vi "Opt3.vi"(0 "Activation Function":enum32{"Sigmoid", "RELU", "Tanh", "Leaky RELU"}(ring), 1 "Weights l+1":dbl[][](array[numeric]), 2 "Weights":dbl[][](array[numeric]), 3 "Biases":dbl[](array[numeric]), 5 "Net Output":dbl[](array[numeric]), 7 "Activations l-1":dbl[](array[numeric]) format="%.2f", 9 "Delta l+1":dbl[](array[numeric]), 12 "Weight Regularizers":enum32{"None", "L1", "L2"}(radio), 13 "Adam Data In":T1) -> (6 "Updated Weights":dbl[][](array[numeric]), 8 "Updated Biases":dbl[](array[numeric]), 14 "Adam Data Out":T1)   [LabVIEW 2019]
uses:
  Iteration Counter.vi
  <vilib>/Analysis/NI_AALBase.lvlib
  <vilib>/Analysis/Matrix/NI_Matrix.lvlib
  <vilib>/Analysis/Matrix/Numeric/Conversions/Matrix To Array - RM.vi
  <vilib>/Analysis/baseanly.llb/Real Outer Product.vi
  <vilib>/Analysis/baseanly.llb/A x Vector.vi
  Adam_data.ctl
panel:
  out "Grad. w":dbl[][](array[numeric])
  out "Grad. b":dbl[](array[numeric])
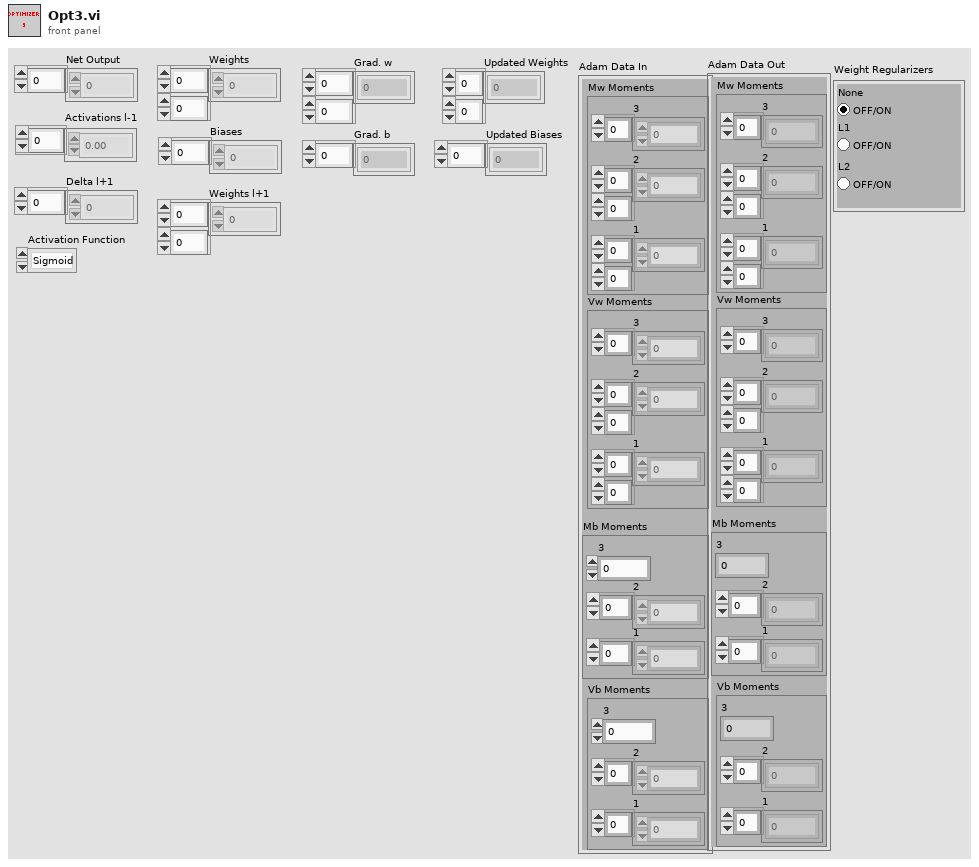
[diagram p1: front panel]
types:
  T1 = typedef "Adam_data.ctl" = cluster{"Mw Moments":cluster{"3 ":dbl[], "2":dbl[][], "1":dbl[][]}, "Vw Moments":cluster{"3":dbl[], "2":dbl[][], "1":dbl[][]}, "Mb Moments":cluster{"3":dbl, "2":dbl[], "1":dbl[]}, "Vb Moments":cluster{"3":dbl, "2":dbl[], "1":dbl[]}}
  T2 = typedef "NI_Matrix.lvlib/RealMatrix.ctl" = dbl[][]
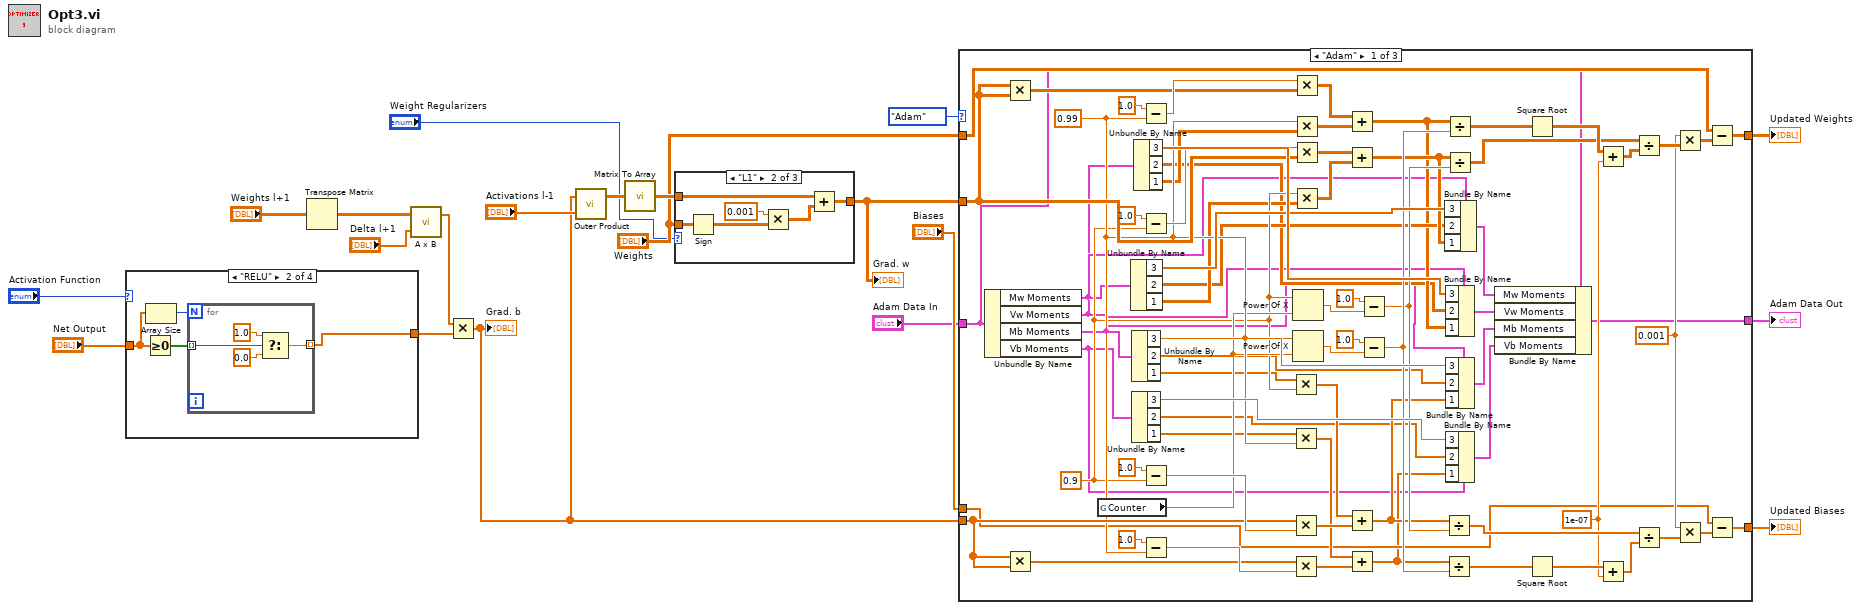
[diagram p0: block diagram]
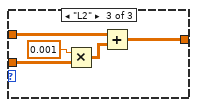
[diagram p3: hidden frame]
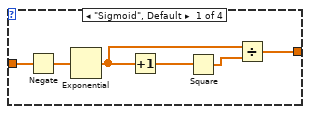
[diagram p6: hidden frame]
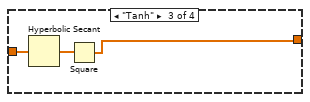
[diagram p7: hidden frame]
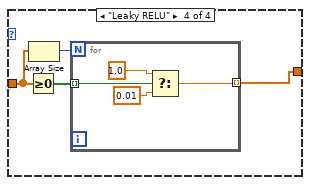
[diagram p8: hidden frame]
diagram:
  n1 = case shown="\"RELU\"" "Activation Function" {
    tunnel: "Net Output" -> [w22 w28 w36 w39]
    tunnel: [w21 w30 w35 w41] -> w19
    frame "Sigmoid", Default {
      n2 = Negate(x=w22) -> (-x=w26:dbl[])
      n3 = Exponential(1:w26) -> (0:w23:dbl[])
      n4 = Increment(x=w23) -> (x+1=w25:dbl[])
      n5 = Square(x=w25) -> (x^2=w24:dbl[])
      n6 = Divide(x=w23, y=w24) -> (x/y=w21:dbl[])
    }
    frame "RELU" {
      n7 = Greater Or Equal To 0?(x=w28) -> (x >= 0?=w29:bool[])
      n8 = Array Size(array=w28) -> (size(s)=w27:i32)
      n9 = for {
        N: w27 -> [_]
        tunnel: [w34] -> w30 mode=indexing
        tunnel: w29 -> [w31] mode=indexing
        n10 = Select(t=1.0, s=w31, f=0.0) -> (s? t:f=w34:dbl)
      }
    }
    frame "Tanh" {
      n11 = Hyperbolic Secant(1:w36) -> (0:w37:dbl[])
      n12 = Square(x=w37) -> (x^2=w35:dbl[])
    }
    frame "Leaky RELU" {
      n13 = Greater Or Equal To 0?(x=w39) -> (x >= 0?=w40:bool[])
      n14 = Array Size(array=w39) -> (size(s)=w38:i32)
      n15 = for {
        N: w38 -> [_]
        tunnel: [w43] -> w41 mode=indexing
        tunnel: w40 -> [w42] mode=indexing
        n16 = Select(t=1.0, s=w42, f=0.01) -> (s? t:f=w43:dbl)
      }
    }
  }
  n17 = Transpose Matrix(1:"Weights l+1") -> (0:w16:dbl[][])
  n18 = call-poly <vilib>:"A x B.vi"("Vector"="Delta l+1", "A"=w16) -> ("A x Vector"=w14:dbl[])  [unwired: 1 out]
  n19 = Multiply(x=w14, y=w19) -> (x*y=w12:dbl[])
  "Grad. b" <- w12
  n20 = call-poly <vilib>:"Outer Product.vi"("Y Vector"="Activations l-1", "X Vector"=w12) -> ("Outer Product"=w11:T2)  [unwired: 1 out]
  n21 = call-poly <vilib>:"Matrix To Array.vi"("Real Matrix"=w11) -> ("Real 2D Array"=w4:dbl[][])
  n22 = case shown="\"L1\"" "Weight Regularizers" {
    tunnel: w4 -> [w46 w48 w57]
    tunnel: [w46 w47 w53] -> w2
    tunnel: "Weights" -> [_ w51 w55]
    frame "None", Default {
    }
    frame "L1" {
      n23 = Sign(1:w51) -> (0:w50:dbl[][])
      n24 = Multiply(x=0.001, y=w50) -> (x*y=w49:dbl[][])
      n25 = Add(x=w48, y=w49) -> (x+y=w47:dbl[][])
    }
    frame "L2" {
      n26 = Multiply(x=0.001, y=w55) -> (x*y=w54:dbl[][])
      n27 = Add(x=w57, y=w54) -> (x+y=w53:dbl[][])
    }
  }
  "Grad. w" <- w2
  n28 = case shown="\"Adam\"" enum16{"Adagrad", "Adadelta", "Adam"}."Adam" ("Optimizer") {
    tunnel: "Weights" -> [w81 w133 w136]
    tunnel: [w80 w133 w136] -> w10
    tunnel: "Biases" -> [w84 w132 w135]
    tunnel: [w83 w132 w135] -> w17
    tunnel: w12 -> [w122 _ _]
    tunnel: w2 -> [w109 _ _]
    tunnel: "Adam Data In" -> [w63 w131 w134]
    tunnel: [w58 w131 w134] -> w6
    frame "Adam" {
      w90 = 1e-07
      w86 = 0.001
      w106 = 0.99
      w102 = 0.9
      n29 = Unbundle By Name(w63) -> ("Mw Moments"=w65:cluster{"3 ":dbl[], "2":dbl[][], "1":dbl[][]}, "Vw Moments"=w64:cluster{"3":dbl[], "2":dbl[][], "1":dbl[][]}, "Mb Moments"=w67:cluster{"3":dbl, "2":dbl[], "1":dbl[]}, "Vb Moments"=w66:cluster{"3":dbl, "2":dbl[], "1":dbl[]})
      n30 = Multiply(x=w109, y=w109) -> (x*y=w112:dbl[][])
      n31 = Multiply(x=w122, y=w122) -> (x*y=w121:dbl[])
      n32 = global read "Iteration Counter.vi" "Counter"() -> (w103:dbl)
      n33 = Unbundle By Name(w65) -> ("3"=w117:dbl[], "2"=w71:dbl[][], "1"=w73:dbl[][])
      n34 = Unbundle By Name(w67) -> ("3"=w129:dbl, "2"=w77:dbl[], "1"=w79:dbl[])
      n35 = Unbundle By Name(w66) -> ("3"=w130:dbl, "2"=w75:dbl[], "1"=w76:dbl[])
      n36 = Unbundle By Name(w64) -> ("3"=w118:dbl[], "2"=w68:dbl[][], "1"=w70:dbl[][])
      n37 = Subtract(x=1.0, y=w106) -> (x-y=w115:dbl)
      n38 = Subtract(x=1.0, y=w102) -> (x-y=w110:dbl)
      n39 = Subtract(x=1.0, y=w102) -> (x-y=w127:dbl)
      n40 = Subtract(x=1.0, y=w106) -> (x-y=w123:dbl)
      n41 = Multiply(x=w79, y=w102) -> (x*y=w126:dbl[])
      n42 = Multiply(x=w76, y=w106) -> (x*y=w120:dbl[])
      n43 = Multiply(x=w122, y=w127) -> (x*y=w125:dbl[])
      n44 = Multiply(x=w121, y=w123) -> (x*y=w119:dbl[])
      n45 = Multiply ("Multiply.vi")(x=w115, y=w112) -> (x*y=w114:dbl[][])
      n46 = Multiply(x=w106, y=w70) -> (x*y=w113:dbl[][])
      n47 = Multiply(x=w110, y=w109) -> (x*y=w108:dbl[][])
      n48 = Multiply(x=w102, y=w73) -> (x*y=w107:dbl[][])
      n49 = Power Of X(1:w103, 2:w102) -> (0:w100:dbl)
      n50 = Power Of X(1:w103, 2:w106) -> (0:w105:dbl)
      n51 = Add(x=w114, y=w113) -> (x+y=w69:dbl[][])
      n52 = Add(x=w108, y=w107) -> (x+y=w72:dbl[][])
      n53 = Add(x=w126, y=w125) -> (x+y=w78:dbl[])
      n54 = Add(x=w120, y=w119) -> (x+y=w74:dbl[])
      n55 = Subtract(x=1.0, y=w100) -> (x-y=w98:dbl)
      n56 = Subtract(x=1.0, y=w105) -> (x-y=w99:dbl)
      n57 = Divide(x=w78, y=w98) -> (x/y=w94:dbl[])
      n58 = Divide(x=w74, y=w99) -> (x/y=w97:dbl[])
      n59 = Divide(x=w69, y=w99) -> (x/y=w92:dbl[][])
      n60 = Divide(x=w72, y=w98) -> (x/y=w89:dbl[][])
      n61 = Bundle By Name(cluster=w65, "3"=w117, "2"=w71, "1"=w72) -> (w62:cluster{"3 ":dbl[], "2":dbl[][], "1":dbl[][]})
      n62 = Bundle By Name(cluster=w64, "3"=w118, "2"=w68, "1"=w69) -> (w61:cluster{"3":dbl[], "2":dbl[][], "1":dbl[][]})
      n63 = Bundle By Name(cluster=w67, "3"=w129, "2"=w77, "1"=w78) -> (w60:cluster{"3":dbl, "2":dbl[], "1":dbl[]})
      n64 = Bundle By Name(cluster=w66, "3"=w130, "2"=w75, "1"=w74) -> (w59:cluster{"3":dbl, "2":dbl[], "1":dbl[]})
      n65 = Bundle By Name(cluster=w63, "Mw Moments"=w62, "Vw Moments"=w61, "Mb Moments"=w60, "Vb Moments"=w59) -> (w58:T1)
      n66 = Square Root(x=w92) -> (sqrt(x)=w91:dbl[][])
      n67 = Square Root(x=w97) -> (sqrt(x)=w96:dbl[])
      n68 = Add(x=w91, y=w90) -> (x+y=w88:dbl[][])
      n69 = Add(x=w96, y=w90) -> (x+y=w95:dbl[])
      n70 = Divide(x=w89, y=w88) -> (x/y=w87:dbl[][])
      n71 = Divide(x=w94, y=w95) -> (x/y=w93:dbl[])
      n72 = Multiply(x=w86, y=w87) -> (x*y=w82:dbl[][])
      n73 = Multiply(x=w86, y=w93) -> (x*y=w85:dbl[])
      n74 = Subtract(x=w81, y=w82) -> (x-y=w80:dbl[][])
      n75 = Subtract(x=w84, y=w85) -> (x-y=w83:dbl[])
    }
    frame "Adadelta" {
    }
    frame "Adagrad" {
    }
  }
  "Updated Biases" <- w17
  "Updated Weights" <- w10
  "Adam Data Out" <- w6
